vi "EtherCAT.vi"() -> (0 "error IO":errorcluster)   [LabVIEW 2020]
uses:
  <resource>/objmgr/IndComECAT.rc
panel:
  out "Slave State 2":u32(ring) items=["UNKNOWN"=0, "Init"=1, "PreOP"=2, "BootStrap"=3, "SafeOP"=4, "OP"=8]
  out "Slave State":u32(ring) items=["UNKNOWN"=0, "Init"=1, "PreOP"=2, "BootStrap"=3, "SafeOP"=4, "OP"=8]
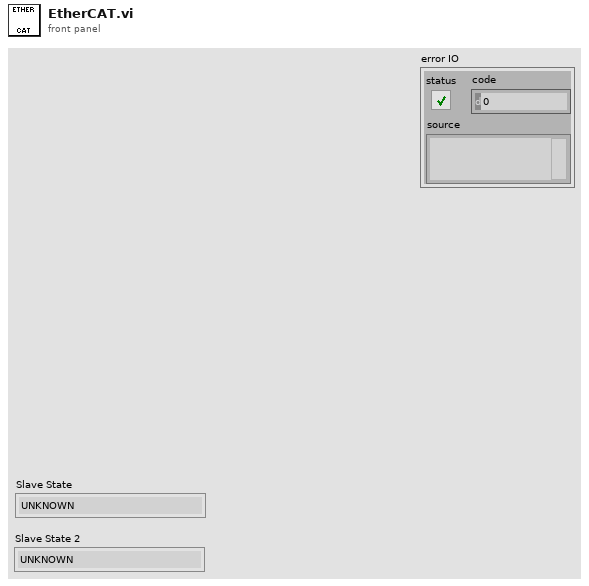
[diagram p1: front panel]
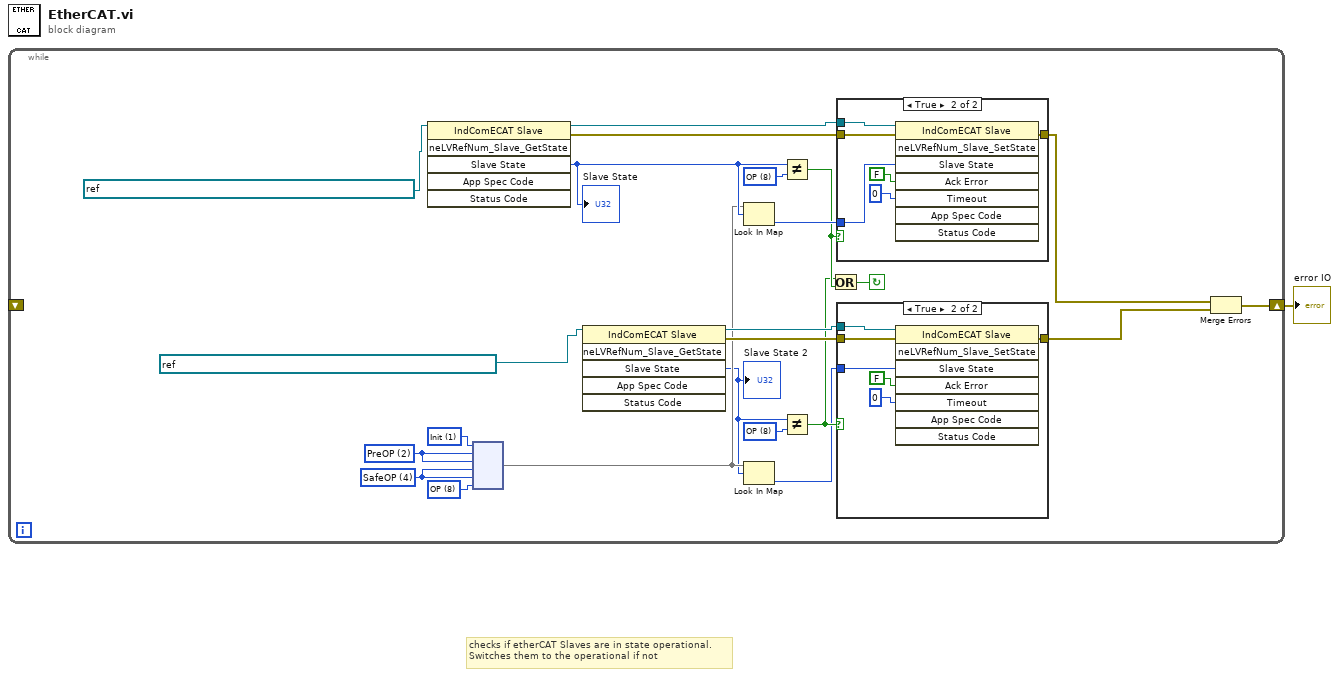
[diagram p0: block diagram]
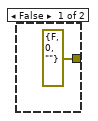
[diagram p2: hidden frame]
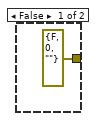
[diagram p3: hidden frame]
diagram:
  # "checks if etherCAT Slaves are in state operational. \nSwitches them to the operational if not"
  n1 = while {
    shift-right: [w4] -> w1
    shift-left: _ -> [_]
    stop <- w10 continue-if-true
    w15 = u32 8 items=["UNKNOWN"=0, "Init"=1, "PreOP"=2, "BootStrap"=3, "SafeOP"=4, "OP"=8] ("Slave State")
    w16 = u32 8 items=["Init"=1, "PreOP"=2, "BootStrap"=3, "SafeOP"=4, "OP"=8] ("Slave State")
    w17 = u32 4 items=["Init"=1, "PreOP"=2, "BootStrap"=3, "SafeOP"=4, "OP"=8] ("Slave State")
    w20 = u32 2 items=["Init"=1, "PreOP"=2, "BootStrap"=3, "SafeOP"=4, "OP"=8] ("Slave State")
    w21 = u32 1 items=["Init"=1, "PreOP"=2, "BootStrap"=3, "SafeOP"=4, "OP"=8] ("Slave State")
    w24 = u32 8 items=["UNKNOWN"=0, "Init"=1, "PreOP"=2, "BootStrap"=3, "SafeOP"=4, "OP"=8] ("Slave State")
    n2 = invoke class="IndComECAT Slave" method="neLVRefNum_Slave_GetState"(reference=refnum<k21> "ni.var.io://ni-crio-9045-01f88613/EtherCAT Master/Device" ("Slave Constant")) -> (reference out=w23:refnum<k21>, error out=w22:errorcluster, "Slave State"=w19:u32)  [unwired: 5 in, 3 out]
    "Slave State" <- w19
    n3 = node(w21, w20, w20, w17, w17, w16) -> (w9:map{u32, u32})
    n4 = invoke class="IndComECAT Slave" method="neLVRefNum_Slave_GetState"(reference=refnum<k21> "ni.var.io://ni-crio-9045-01f88613/EtherCAT Master/Device2" ("Slave Constant")) -> (reference out=w14:refnum<k21>, error out=w13:errorcluster, "Slave State"=w8:u32)  [unwired: 5 in, 3 out]
    "Slave State 2" <- w8
    n5 = Look In Map(map=w9, key=w19) -> (value=w18:u32)  [unwired: 1 in, 1 out]
    n6 = Look In Map(map=w9, key=w8) -> (value=w7:u32)  [unwired: 1 in, 1 out]
    n7 = Not Equal?(x=w19, y=w24) -> (x != y?=w12:bool)
    n8 = Not Equal?(x=w8, y=w15) -> (x != y?=w11:bool)
    n9 = Or(x=w11, y=w12) -> (x .or. y?=w10:bool)
    n10 = case shown="True" w12 {
      tunnel: w23 -> [_ w38]
      tunnel: w22 -> [_ w37]
      tunnel: w18 -> [_ w34]
      tunnel: [errorcluster {"status"=FALSE, "code"=0, "source"=""} ("error out") w33] -> w6
      frame False {
      }
      frame True {
        n11 = invoke class="IndComECAT Slave" method="neLVRefNum_Slave_SetState"(reference=w38, error in=w37, "Slave State"=w34, "Ack Error"=FALSE, "Timeout"=u32 0) -> (error out=w33:errorcluster)  [unwired: 3 in, 7 out]
      }
    }
    n12 = case shown="True" w11 {
      tunnel: w14 -> [_ w31]
      tunnel: w13 -> [_ w30]
      tunnel: w7 -> [_ w27]
      tunnel: [errorcluster {"status"=FALSE, "code"=0, "source"=""} ("error out") w26] -> w5
      frame False {
      }
      frame True {
        n13 = invoke class="IndComECAT Slave" method="neLVRefNum_Slave_SetState"(reference=w31, error in=w30, "Slave State"=w27, "Ack Error"=FALSE, "Timeout"=u32 0) -> (error out=w26:errorcluster)  [unwired: 3 in, 7 out]
      }
    }
    n14 = Merge Errors(w6, w5) -> (w4:errorcluster)
  }
  "error IO" <- w1
